vi "scan and load params.vi"() -> (0 "Level":bool, 1 "RFOnB2":bool, 2 "RFOnA2":bool, 3 "Serial Port Select":refnum<visa-resource-name>="COM3", 4 "POWER dBm B":dbl min=-100.0 max=24.0 step=1.0 format="%.2g", 5 "POWER dBm A":dbl min=-100.0 max=24.0 step=1.0 format="%.2g", 6 "Level B 2":bool, 7 "Level A 2":bool, 8 "RF  FREQUENCY MHz  B":dbl=1000.0 min=54.0 max=13900.0 step=1.0 format="%.7g", 9 "RF  FREQUENCY MHz A":dbl=1000.0 min=54.0 max=13900.0 step=1.0 format="%.7g")   [LabVIEW 2012]
panel:
  in  "POWER dBm":dbl min=-75.0 max=20.0 step=1.0 format="%.2g"
  in  "RF  FREQUENCY MHz":dbl=1000.0 min=53.0 max=13999.999 step=1.0 format="%.7g"
  out "Device Under Control":string
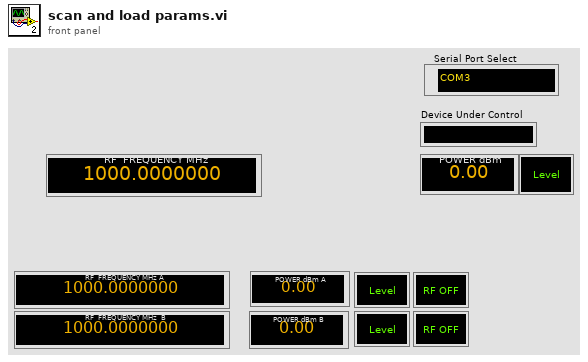
[diagram p1: front panel]
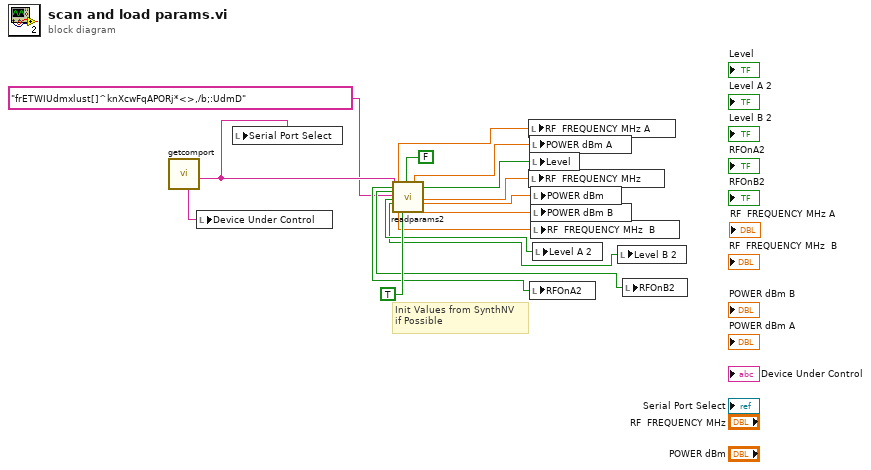
[diagram p0: block diagram]
diagram:
  # "Init Values from SynthNV\nif Possible"
  n1 = call "getcomport.vi"() -> ("Port"=w2:string, "Device"=w16:string)  [unwired: 9 in, 1 out]
  n2 = local write "Device Under Control"(w16) -> ()
  n3 = local write "Serial Port Select"(w2) -> ()
  n4 = call "readparams2.vi"("Port In"=w2, "var query"="frETWIUdmxlust[]^knXcwFqAPORj*<>,/b;:UdmD", "Get F&A"=TRUE, "Prog Chan?"=FALSE) -> ("RFonA"=w4:bool, "RFonB"=w3:bool, "LevA"=w6:bool, "LevB"=w5:bool, "FchA"=w14:dbl, "FchB"=w11:dbl, "AdBm"=w13:dbl, "BdBm"=w12:dbl, "NowLevel"=w10:bool, "NowFreq"=w7:dbl, "NowdBm"=w9:dbl)  [unwired: 9 in, 4 out]
  n5 = local write "RF  FREQUENCY MHz A"(w14) -> ()
  n6 = local write "RF  FREQUENCY MHz"(w7) -> ()
  n7 = local write "POWER dBm A"(w13) -> ()
  n8 = local write "Level"(w10) -> ()
  n9 = local write "RFOnA2"(w4) -> ()
  n10 = local write "POWER dBm"(w9) -> ()
  n11 = local write "POWER dBm B"(w12) -> ()
  n12 = local write "RF  FREQUENCY MHz  B"(w11) -> ()
  n13 = local write "Level A 2"(w6) -> ()
  n14 = local write "Level B 2"(w5) -> ()
  n15 = local write "RFOnB2"(w3) -> ()
